vi "Read Registry Value STR.vi"(8 "error in (no error)":errorcluster, 9 "default data":string, 10 "value":string, 11 "refnum":T1) -> (0 "error out":errorcluster, 1 "String/Binary data":string, 2 "data type":T2(ring), 3 "refnum out":T1)   [LabVIEW 2020]
doc: "Reads data and data type from value. If the key or value does not exist or an unrecoverable error occurs, the VI returns the default value."
uses:
  Registry refnum.ctl
  Advapi32.dll
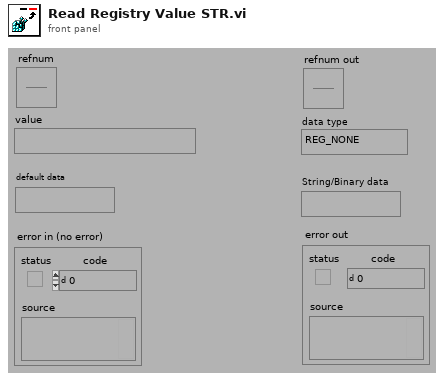
[diagram p1: front panel]
types:
  T1 = typedef "Registry refnum.ctl" = refnum<k1>
  T2 = enum32{"REG_NONE", "REG_SZ", "REG_EXPAND_SZ", "REG_BINARY", "REG_DWORD_LITTLE_ENDIAN", "REG_DWORD_BIG_ENDIAN", "REG_LINK", "REG_MULTI_SZ", "REG_RESOURCE_LIST", "REG_FULL_RESOURCE_DESCRIPTOR", "REG_RESOURCE_REQUIREMENTS_LIST"}
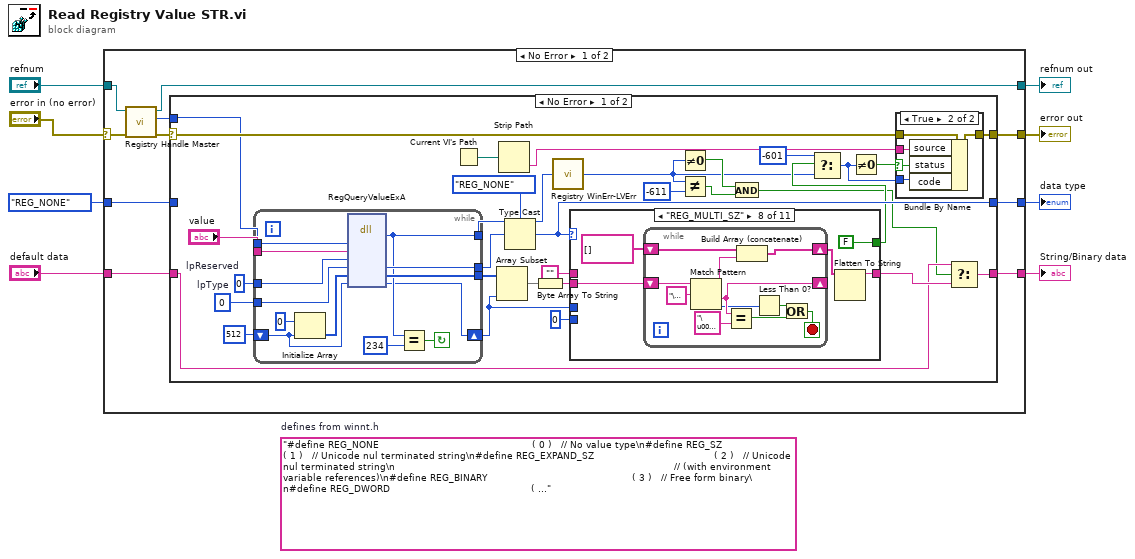
[diagram p0: block diagram]
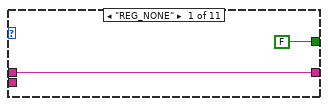
[diagram p3: hidden frame]
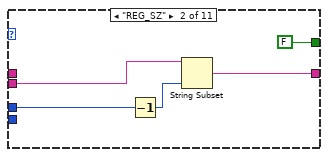
[diagram p4: hidden frame]
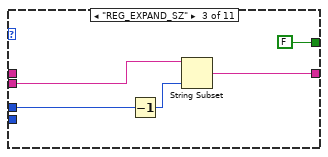
[diagram p5: hidden frame]
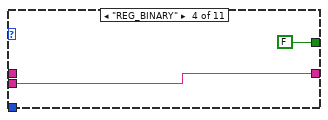
[diagram p6: hidden frame]
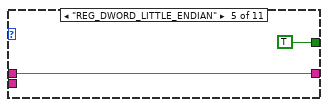
[diagram p7: hidden frame]
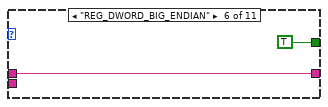
[diagram p8: hidden frame]
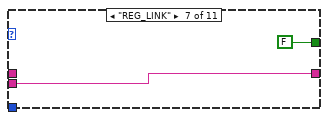
[diagram p9: hidden frame]
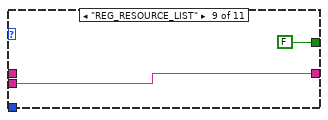
[diagram p10: hidden frame]
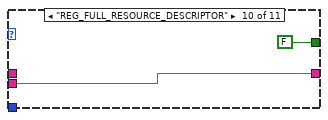
[diagram p11: hidden frame]
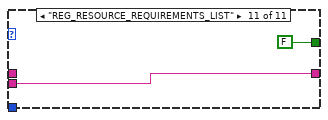
[diagram p12: hidden frame]
diagram:
  (unwired) "#define REG_NONE                                                   ( 0 )   // No value type\n#define REG_SZ                                                        ( 1 )   // Unicode nul terminated string\n#define REG_EXPAND_SZ                                        ( 2 )   // Unicode nul terminated string\n                                                                                             // (with environment variable references)\n#define REG_BINARY                                                ( 3 )   // Free form binary\n#define REG_DWORD                                               ( 4 )   // 32-bit number\n#define REG_DWORD_LITTLE_ENDIAN                  ( 4 )   // 32-bit number (same as REG_DWORD)\n#define REG_DWORD_BIG_ENDIAN                        ( 5 )   // 32-bit number\n#define REG_LINK                                                      ( 6 )   // Symbolic Link (unicode)\n#define REG_MULTI_SZ                                            ( 7 )   // Multiple Unicode strings\n#define REG_RESOURCE_LIST                                ( 8 )   // Resource list in the resource map\n#define REG_FULL_RESOURCE_DESCRIPTOR      ( 9 )   // Resource list in the hardware description\n#define REG_RESOURCE_REQUIREMENTS_LIST ( 10 )\n"  # defines from winnt.h
  n1 = case shown="No Error" "error in (no error)" {
    selector: "error in (no error)" -> [w15 w117]
    tunnel: [w18 w115] -> w7
    tunnel: [w17 w114] -> w8
    tunnel: [w16 w117] -> w6
    tunnel: "refnum" -> [w14 w116]
    tunnel: [w13 w116] -> w3
    tunnel: T2."REG_NONE" -> [w10 w115]
    tunnel: "default data" -> [w9 w114]
    frame No Error {
      n2 = call "Registry Handle Master.vi"("error in (no error)"=w15, "refnum"=w14) -> ("error out"=w12:errorcluster, "key handle out"=w11:u64, "refnum out"=w13:T1)  [unwired: 4 in, 3 out]
      n3 = case shown="No Error" w12 {
        selector: w12 -> [w30 w111]
        tunnel: [w49 w113] -> w18
        tunnel: [w28 w112] -> w17
        tunnel: [w37 w111] -> w16
        tunnel: w11 -> [w29 _]
        tunnel: w10 -> [_ w113]
        tunnel: w9 -> [w26 w112]
        frame No Error {
          w38 = u32 0  # lpType
          w40 = u64 0  # lpReserved
          n4 = while {
            tunnel: [w62] -> w42
            tunnel: [w61] -> w41
            tunnel: w40 -> [w60]
            tunnel: "value" -> [w59]
            tunnel: w38 -> [w57]
            tunnel: [w53] -> w35
            tunnel: w29 -> [w55]
            shift-right: [w50] -> w19
            shift-left: u32 512 -> [w51]
            stop <- w54 continue-if-true
            n5 = Initialize Array(u8 0, w51) -> (w58:u8[])
            n6 = dll-call lib="Advapi32.dll" fn="RegQueryValueExA"("hKey"=w55, "lpValueName"=w59, "lpReserved"=w60, "lpType"=w57, "lpData"=w58, "lpcbData"=w51) -> ("return type"=w53:i32, "lpType"=w61:u32, "lpData"=w62:u8[], "lpcbData"=w50:u32)  [unwired: 3 in, 5 out]
            n7 = Equal?(x=w53, y=234) -> (x = y?=w54:bool)
          }
          n8 = Current VI's Path() -> (path=w44:path)
          n9 = Array Subset(array=w42, length=w19) -> (w43:u8[])  [unwired: 1 in]
          n10 = Strip Path(path=w44) -> (name=w45:string)  [unwired: 1 out]
          n11 = Type Cast(type=T2."REG_NONE", x=w41) -> (*(type *) &x=w49:T2)
          n12 = Byte Array To String(unsigned byte array=w43) -> (string=w36:string)
          n13 = call "Registry WinErr-LVErr.vi"("Windows error"=w35) -> ("LabVIEW error"=w22:i32)  [unwired: 4 out]
          n14 = case shown="\"REG_MULTI_SZ\"" w49 {
            tunnel: w36 -> [_ w74 w79 w82 _ _ w88 w92 w106 w108 w110]
            tunnel: w19 -> [_ w75 w80 _ _ _ _ _ _ _ _]
            tunnel: [w70 w72 w77 w82 w84 w86 w88 w91 w106 w108 w110] -> w27
            tunnel: "" -> [w70 _ _ _ w84 w86 _ _ _ _ _]
            tunnel: u32 0 -> [_ _ _ _ _ _ _ _ _ _ _]
            tunnel: [FALSE FALSE FALSE FALSE TRUE TRUE FALSE FALSE FALSE FALSE FALSE] -> w34
            frame "REG_NONE" {
            }
            frame "REG_SZ" {
              n15 = Decrement(x=w75) -> (x-1=w73:u32)
              n16 = String Subset(string=w74, length (rest)=w73) -> (substring=w72:string)  [unwired: 1 out]
            }
            frame "REG_EXPAND_SZ" {
              n17 = Decrement(x=w80) -> (x-1=w78:u32)
              n18 = String Subset(string=w79, length (rest)=w78) -> (substring=w77:string)  [unwired: 1 out]
            }
            frame "REG_BINARY" {
            }
            frame "REG_DWORD_LITTLE_ENDIAN" {
            }
            frame "REG_DWORD_BIG_ENDIAN" {
            }
            frame "REG_LINK" {
            }
            frame "REG_MULTI_SZ" {
              n19 = while {
                shift-right: [w98] -> _
                shift-left: w92 -> [w103]
                shift-right: [w99] -> w89
                shift-left: string[] [] -> [w101]
                stop <- w94 stop-if-true
                n20 = Match Pattern(string=w103, regular expression="\u0000") -> (before substring=w100:string, after substring=w98:string, offset past match=w97:i32)  [unwired: 2 out]
                n21 = Equal?(x=w98, y="\u0000") -> (x = y?=w95:bool)
                n22 = Build Array (concatenate)(w101, w100) -> (w99:string[])
                n23 = Less Than 0?(x=w97) -> (x < 0?=w96:bool)
                n24 = Or(x=w96, y=w95) -> (x .or. y?=w94:bool)
              }
              n25 = Flatten To String(anything=w89) -> (data string=w91:string)  [unwired: 1 in, 4 out]
            }
            frame "REG_RESOURCE_LIST" {
            }
            frame "REG_FULL_RESOURCE_DESCRIPTOR" {
            }
            frame "REG_RESOURCE_REQUIREMENTS_LIST" {
            }
          }
          n26 = Not Equal To 0?(x=w22) -> (x != 0?=w23:bool)
          n27 = Not Equal?(x=w22, y=-611) -> (x != y?=w24:bool)
          n28 = And(x=w23, y=w24) -> (x .and. y?=w21:bool)
          n29 = Select(t=-601, s=w34, f=w22) -> (s? t:f=w32:i32)
          n30 = Not Equal To 0?(x=w32) -> (x != 0?=w31:bool)
          n31 = case shown="True" w31 {
            selector: w31 -> [_ w64]
            tunnel: w45 -> [_ w68]
            tunnel: [w63 w67] -> w37
            tunnel: w32 -> [_ w66]
            tunnel: w30 -> [w63 w65]
            frame False {
            }
            frame True {
              n32 = Bundle By Name(cluster=w65, "source"=w68, "status"=w64, "code"=w66) -> (w67:errorcluster)
            }
          }
          n33 = Select(t=w26, s=w21, f=w27) -> (s? t:f=w28:string)
        }
        frame Error {
        }
      }
    }
    frame Error {
    }
  }
  "error out" <- w6
  "String/Binary data" <- w8
  "data type" <- w7
  "refnum out" <- w3
